vi "QMH_Create_ICR_Queue.vi"(8 "error in (no error)":errorcluster caption="entrée d'erreur (pas d'erreur)") -> (0 "error out":errorcluster caption="sortie d'erreur", 3 "ICR Queue":refnum<queue>)   [LabVIEW 2015]
uses:
  controls/QMH_ICR_Message.ctl
  controls/QMH_ICR_Command.ctl
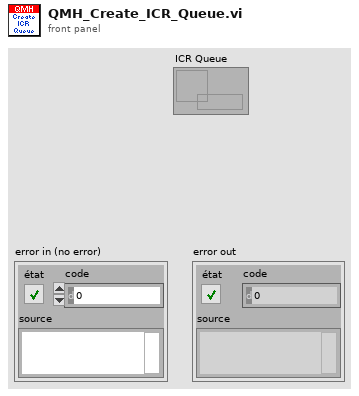
[diagram p1: front panel]
types:
  T1 = typedef "QMH_ICR_Command.ctl" = enum16{"Initialize", "Hardware Setup", "Waiting for Trigger", "Sequence Started", "Sequence Finished", "Writing Data", "Hardware Reset", "Exit"}
  T2 = typedef "QMH_ICR_Message.ctl" = cluster{"Command":T1, "Data":variant}
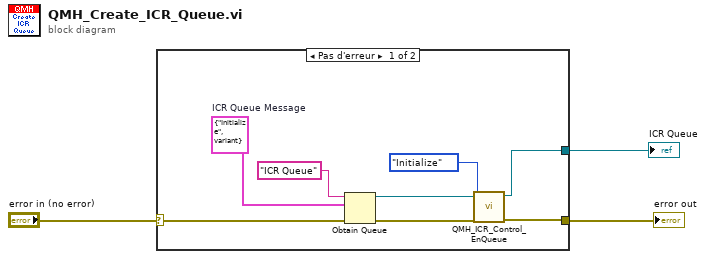
[diagram p0: block diagram]
diagram:
  n1 = case shown="Pas d'erreur" "error in (no error)" {
    selector: "error in (no error)" -> [w10 w12]
    tunnel: [w7 w12] -> w2
    tunnel: [w6 _] -> w1
    frame No Error {
      w9 = T2 {"Command"=enum."Initialize", "Data"=variant}  # ICR Queue Message
      n2 = Obtain Queue(name (unnamed)="ICR Queue" ("nom (aucun)"), element data type=w9, error in (no error)=w10) -> (queue out=w5:refnum<queue>, error out=w8:errorcluster)  [unwired: 2 in, 1 out]
      n3 = call "QMH_ICR_Control_EnQueue.vi"("error in (no error)"=w8, "Command"=QMH_ICR_Command."Initialize", "ICR Queue"=w5) -> ("error out"=w7:errorcluster, "ICR Queue"=w6:refnum<queue>)  [unwired: 7 in]
    }
    frame Error {
    }
  }
  "error out" <- w2
  "ICR Queue" <- w1
